vi "Set calibration factor.vi"(8 "error in (no error)":errorcluster, 10 "Calibration Factor":dbl=-26.67 format="%#5_4g", 11 "VISA resource name":refnum<visa-resource-name>="GPIB0::21::INSTR") -> (0 "error out":errorcluster, 3 "VISA resource name out":refnum<visa-resource-name>)   [LabVIEW 2009]
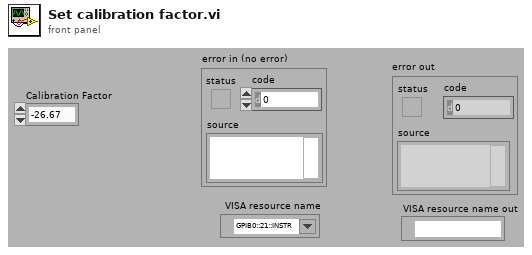
[diagram p1: front panel]
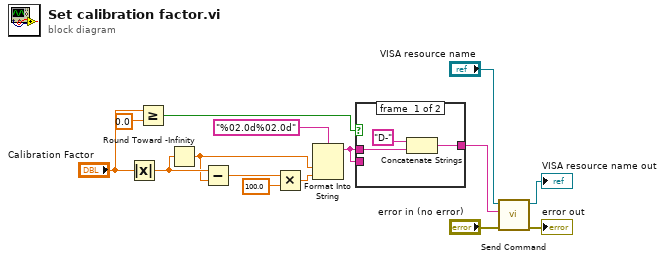
[diagram p0: block diagram]
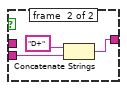
[diagram p2: hidden frame]
diagram:
  n1 = Absolute Value(x="Calibration Factor") -> (abs(x)=w9:dbl)
  n2 = Greater Or Equal?(x="Calibration Factor", y=0.0) -> (x >= y?=w12:bool)
  n3 = Round Toward -Infinity(1:w9) -> (0:w3:dbl)
  n4 = Subtract(x=w9, y=w3) -> (x-y=w8:dbl)
  n5 = Multiply(x=w8, y=100.0) -> (x*y=w6:dbl)
  n6 = Format Into String(format string="%02.0d%02.0d", w3, w6) -> (resulting string=w4:string)  [unwired: 2 in, 1 out]
  n7 = case shown="True" w12 {
    tunnel: [w16 w20] -> w11
    tunnel: w4 -> [_ w19]
    tunnel: w4 -> [w17 _]
    frame #0 {
      n8 = Concatenate Strings("D-" ("string"), w17) -> (w16:string)
    }
    frame #1 {
      n9 = Concatenate Strings("D+" ("string"), w19) -> (w20:string)
    }
  }
  n10 = call "Send Command.vi"("error in (no error)"="error in (no error)", "write buffer"=w11, "VISA resource name"="VISA resource name") -> ("error out"=→"error out":errorcluster, "VISA resource name out"=→"VISA resource name out":refnum<visa-resource-name>)  [unwired: 7 in]
